vi "ColorSensorDemo.vi"() -> ()   [LabVIEW 2011]
uses:
  API/ColorSensorlib.lvlib
panel:
  out "Blue":i32
  out "Green":i32
  out "Red":i32
  in  "端口号":i32
  in  "Quit":bool
  in  "Get":bool
  in  "Init":bool
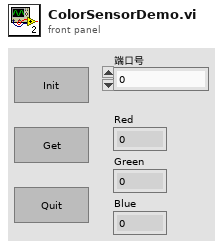
[diagram p1: front panel]
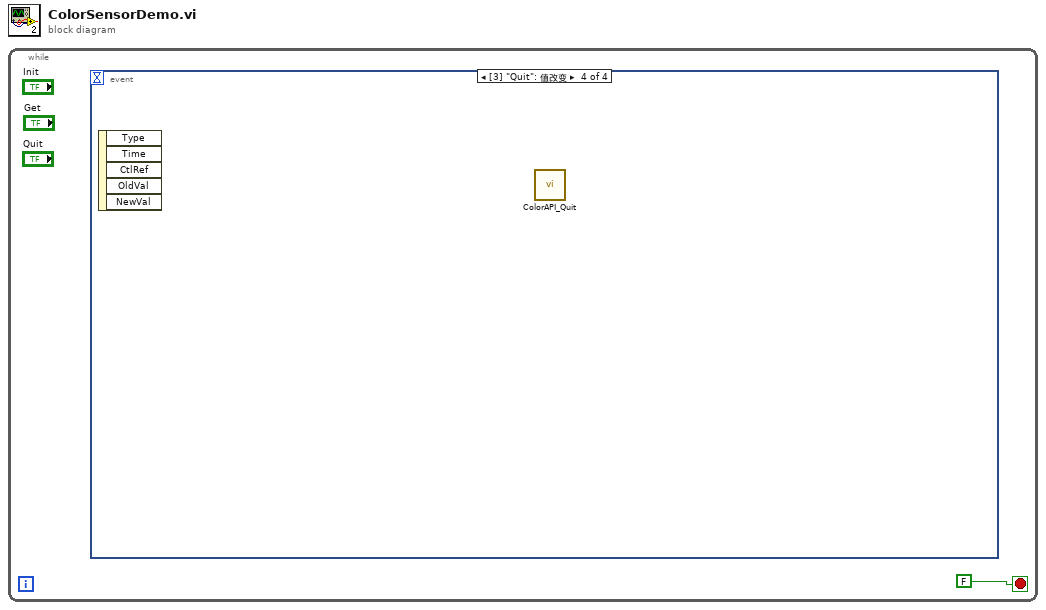
[diagram p0: block diagram]
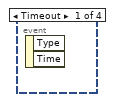
[diagram p2: hidden frame]
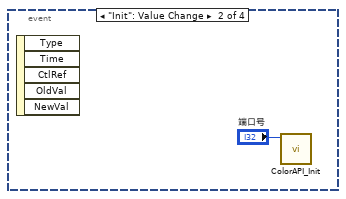
[diagram p3: hidden frame]
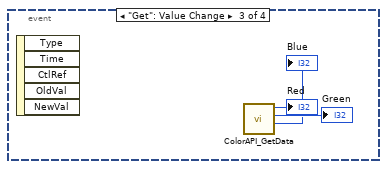
[diagram p4: hidden frame]
diagram:
  n1 = while {
    stop <- FALSE stop-if-true
    n2 = event shown="[3] \"Quit\": 值改变" {
      selector: _ -> [_ _ _ _]
      dyn-events: _ -> [_ _ _ _]
      timeout: _ -> [_ _ _ _]
      event Timeout {
        n3 = event-data() -> ()  [unwired: 1 in, 2 out]
      }
      event "Init": Value Change {
        n4 = event-data() -> ()  [unwired: 1 in, 5 out]
        n5 = call "ColorAPI_Init.vi"("端口号"="端口号") -> ()  [unwired: 8 in, 3 out]
      }
      event "Get": Value Change {
        n6 = event-data() -> ()  [unwired: 1 in, 5 out]
        n7 = call "ColorAPI_GetData.vi"() -> ("Blue"=→"Blue":i32, "Green"=→"Green":i32, "Red"=→"Red":i32)  [unwired: 8 in, 1 out]
      }
      event "Quit": Value Change {
        n8 = event-data() -> ()  [unwired: 1 in, 5 out]
        n9 = call "ColorAPI_Quit.vi"() -> ()  [unwired: 11 in, 1 out]
      }
    }
  }
